vi "Read TCP Connection.vi"(8 "error in (no error)":errorcluster, 11 "MB_TCP_Device in":refnum<class "MB_TCP_Device.lvclass">) -> (0 "error out":errorcluster, 2 "TCP Connection":refnum<k5>, 3 "MB_TCP_Device out":refnum<class "MB_TCP_Device.lvclass">)   [LabVIEW 2023, in "MB_TCP_Device.lvclass"]
uses:
  MB_TCP_Device.lvclass
  MB_TCP_Device.lvclass/MB_TCP_Device.ctl
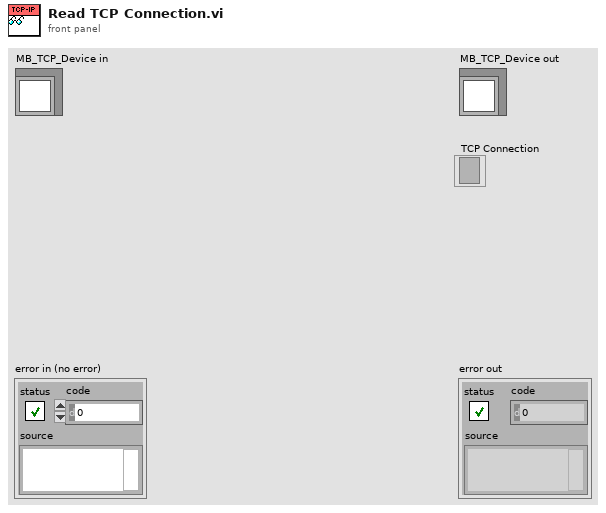
[diagram p1: front panel]
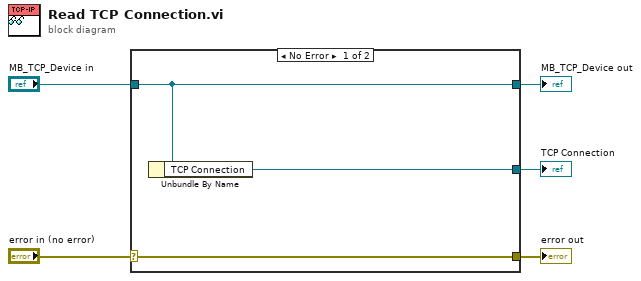
[diagram p0: block diagram]
diagram:
  n1 = case shown="No Error" "error in (no error)" {
    selector: "error in (no error)" -> [w8 w9]
    tunnel: [w8 w9] -> w4
    tunnel: [w7 w10] -> w2
    tunnel: "MB_TCP_Device in" -> [w7 w10]
    tunnel: [w6 _] -> w1
    frame No Error {
      n2 = Unbundle By Name(w7) -> ("TCP Connection"=w6:refnum<k5>)
    }
    frame Error {
    }
  }
  "error out" <- w4
  "MB_TCP_Device out" <- w2
  "TCP Connection" <- w1
